vi "Update Sensor Names.vi"(8 "error in (no error)":errorcluster, 11 "Create Test Channel Model in":refnum<class "Create Test Channel Model.lvclass">) -> (0 "error out":errorcluster, 3 "Create Test Channel Model out":refnum<class "Create Test Channel Model.lvclass">)   [LabVIEW 2013, in "Create Test Channel Model.lvlib" / "Create Test Channel Model.lvclass"]
uses:
  Create Test Channel Model.lvclass
  Create Test Channel Model.lvclass/Create Test Channel Model.ctl
  <vilib>/ActorFrameworkMVC/View Observer/View Registry/View Registry.lvclass/View Registry.ctl
  Create Test Channel Model Messages/Abstract Create Test Channel Sensor Names Msg/Abstract Create Test Channel Sensor Names Msg.lvclass
  <vilib>/ActorFrameworkMVC/View Observer/Data Message/Data Message.lvclass
  <vilib>/ActorFrameworkMVC/View Observer/View Registry/View Registry.lvclass
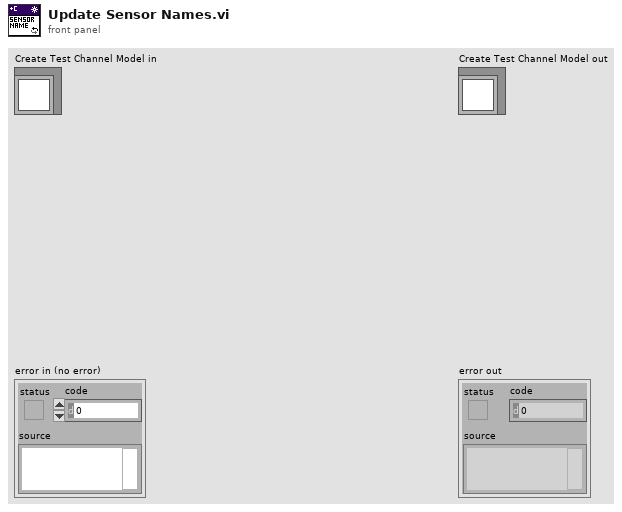
[diagram p1: front panel]
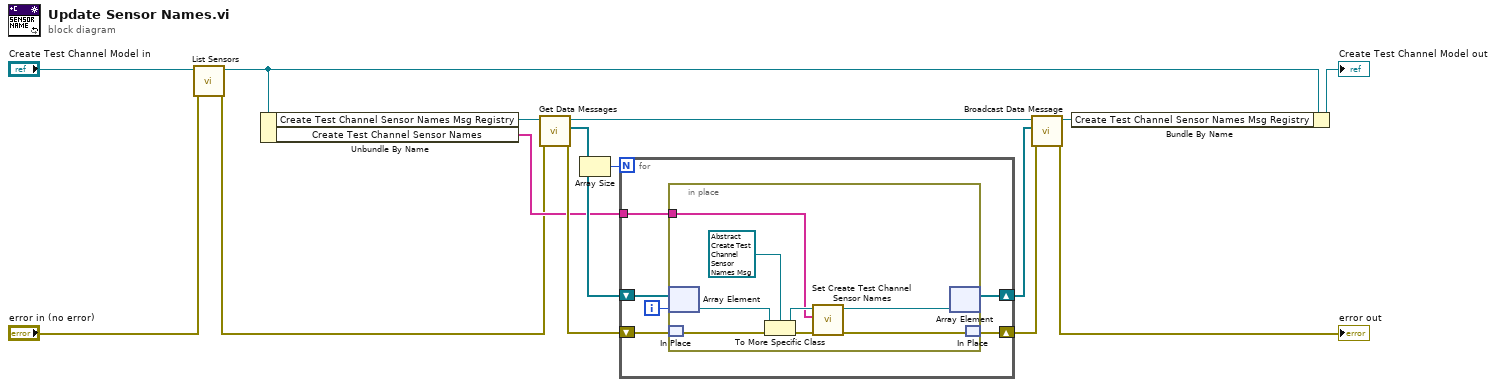
[diagram p0: block diagram]
diagram:
  n1 = call "List Sensors.vi"("error in (no error)"="error in (no error)", "Create Test Channel Model in"="Create Test Channel Model in") -> ("error out"=w1:errorcluster, "Create Test Channel Model out"=w3:refnum<class "Create Test Channel Model.lvclass">)  [unwired: 8 in]
  n2 = Unbundle By Name(w3) -> ("Create Test Channel Sensor Names Msg Registry"=w15:refnum<class "View Registry.lvclass">, "Create Test Channel Sensor Names"=w7:string[])
  n3 = call <vilib>:"Get Data Messages.vi"("error in (no error)"=w1, "View Registry in"=w15) -> ("error out"=w11:errorcluster, "Data Messages"=w12:refnum<class "Data Message.lvclass">[], "View Registry out"=w14:refnum<class "View Registry.lvclass">)  [unwired: 7 in]
  n4 = Array Size(array=w12) -> (size(s)=w13:i32)
  n5 = for {
    N: w13 -> [_]
    shift-right: [w20] -> w10
    shift-left: w12 -> [w21]
    shift-right: [w17] -> w9
    shift-left: w11 -> [w19]
    tunnel: w7 -> [w18]
    i -> [w16]
    n6 = in-place {
      in-place-border: w18 -> [w22]
      n7 = in-place-array #1(w21, w16) -> (w27:refnum<class "Data Message.lvclass">)
      n8 = in-place-match #2(w19) -> (w29:errorcluster)
      n9 = To More Specific Class(target class=refnum<class "Abstract Create Test Channel Sensor Names Msg.lvclass"> refnum ("Create Test Channel Model.lvlib:Abstract Create Test Channel Sensor Names Msg.lvclass"), reference=w27, error in=w29) -> (specific class reference=w23:refnum<class "Abstract Create Test Channel Sensor Names Msg.lvclass">, error out=w26:errorcluster)
      n10 = call "Set Create Test Channel Sensor Names.vi"("error in (no error)"=w26, "Create Test Channel Sensor Names"=w22, "Abstract Create Test Channel Sensor Names Msg in"=w23) -> ("error out"=w25:errorcluster, "Abstract Create Test Channel Sensor Names Msg out"=w24:refnum<class "Abstract Create Test Channel Sensor Names Msg.lvclass">)  [unwired: 7 in]
      n11 = in-place-array #1(w24) -> (w20:refnum<class "Data Message.lvclass">[])  [unwired: 1 out]
      n12 = in-place-match #2(w25) -> (w17:errorcluster)
    }
  }
  n13 = call <vilib>:"Broadcast Data Message.vi"("error in (no error)"=w9, "Data Messages"=w10, "View Registry in"=w14) -> ("error out"=→"error out":errorcluster, "View Registry out"=w8:refnum<class "View Registry.lvclass">)  [unwired: 7 in]
  n14 = Bundle By Name(cluster=w3, "Create Test Channel Sensor Names Msg Registry"=w8) -> (→"Create Test Channel Model out":refnum<class "Create Test Channel Model.lvclass">)
